vi "Find Path.vi"(8 "error in":errorcluster, 9 "end":string, 10 "start":string, 11 "FlexWorktable in":refnum<class "FlexWorktable.lvclass">) -> (0 "error out":errorcluster, 1 "Point Names":string[](array[string]), 2 "Points":refnum<class "Vec3d.lvclass">[](array[class]), 3 "FlexWorktable out":refnum<class "FlexWorktable.lvclass">)   [LabVIEW 2024]
uses:
  Vec3d Class/Vec3d.lvclass
  FlexWorktable/FlexWorktable.lvclass
  Node.ctl
  fd1d9aa2-fa2c-4f05-b8b8-dc46fe165a2d.vi
  c3290523-0369-4e35-a41e-cda71a30bf11.vi
  852f93a0-a655-4212-b043-5cd013f93269.vi
  5b83d3e8-932b-40b1-bf24-38bcf14b1dea.vi
  <vilib>/Comparison/Equal/Equal Functor/Equal Functor.lvclass
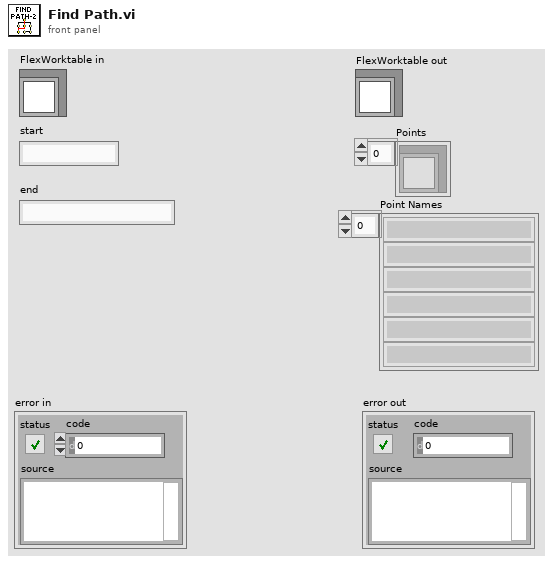
[diagram p1: front panel]
types:
  T1 = typedef "Node.ctl" = cluster{"distance":dbl, "visited":bool, "path to":i32[], "neighbors":i32[], "name":string, "id":i32}
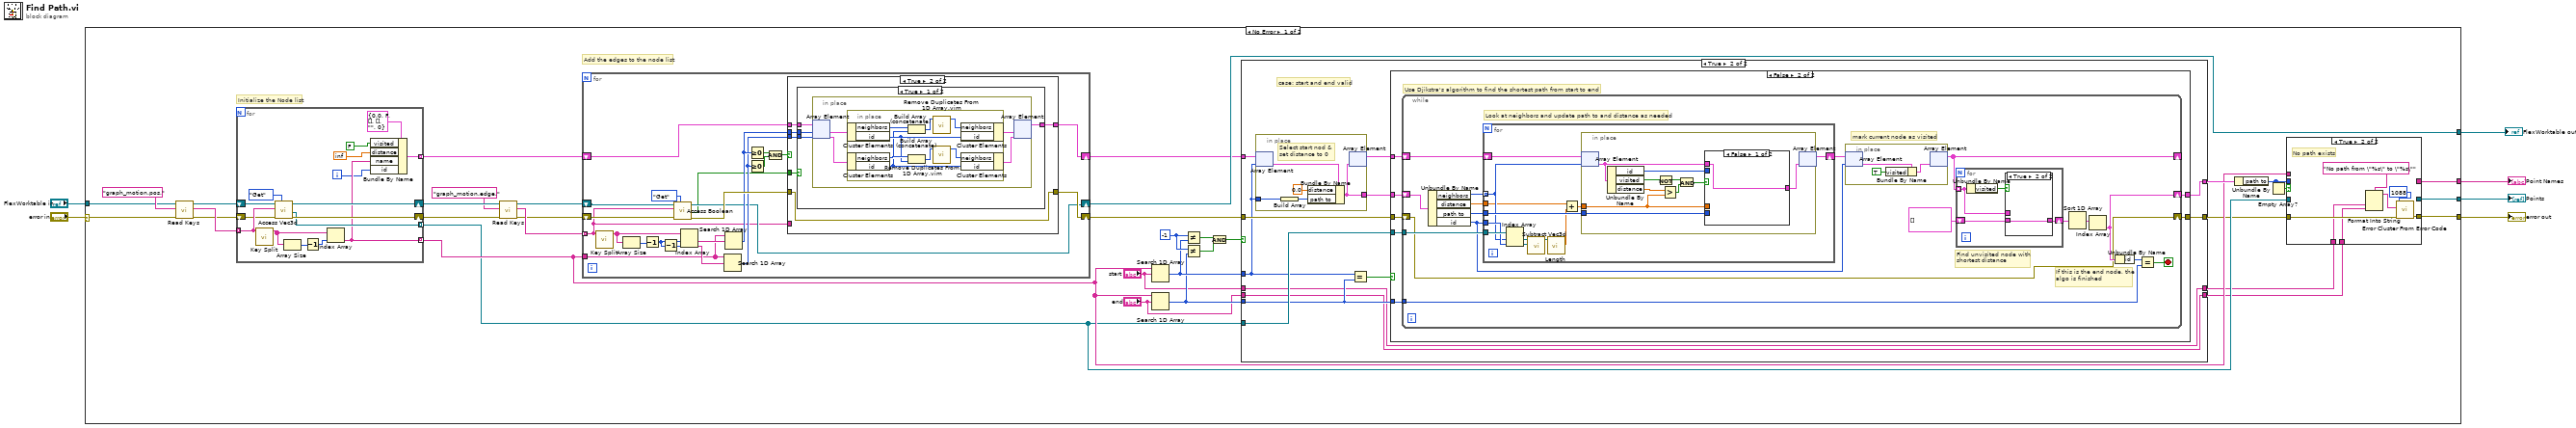
[diagram p0: block diagram]
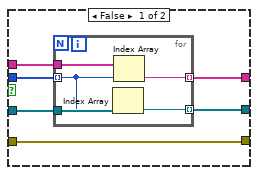
[diagram p2: hidden frame]
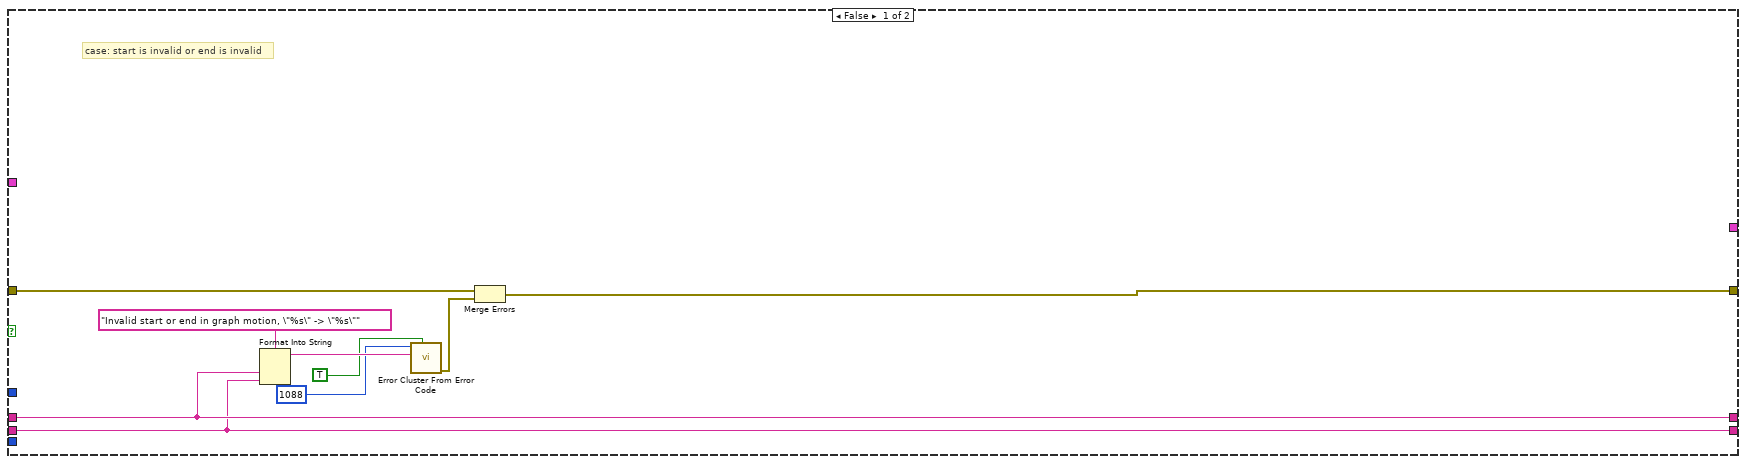
[diagram p3: hidden frame]
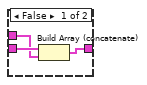
[diagram p5: hidden frame]
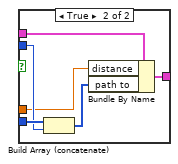
[diagram p6: hidden frame]
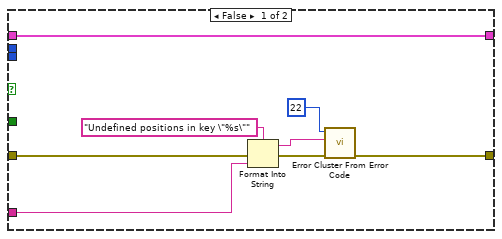
[diagram p7: hidden frame]
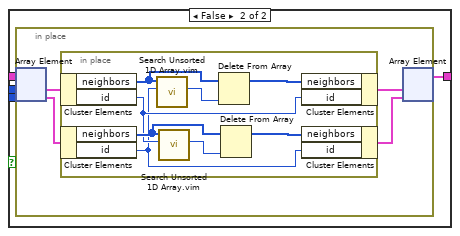
[diagram p8: hidden frame]
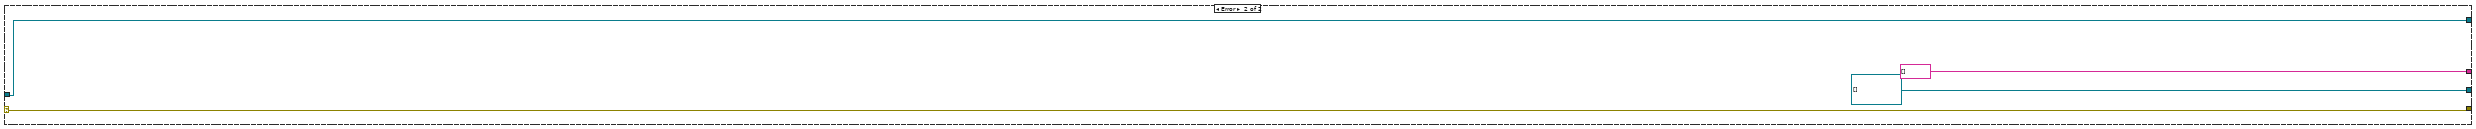
[diagram p9: hidden frame]
diagram:
  n1 = case shown="No Error" "error in" {
    selector: "error in" -> [w15 w238]
    tunnel: [w19 string[] []] -> w6
    tunnel: [w18 refnum<class "Vec3d.lvclass">[] []] -> w5
    tunnel: [w9 w238] -> w4
    tunnel: [w17 w239] -> w3
    tunnel: "FlexWorktable in" -> [w16 w239]
    frame No Error {
      w30 = -1
      # "Add the edges to the node list"
      # "Initialize the Node list"
      n2 = call-dynamic "Read Keys.vi"("error in (no error)"=w15, "Selector"="graph_motion.pos.", "FlexWorktable in"=w16) -> ("error out"=w38:errorcluster, "Keys"=w40:string[], "FlexWorktable out"=w39:refnum<class "FlexWorktable.lvclass">)  [unwired: 6 in]
      n3 = for {
        tunnel: w40 -> [w231] mode=indexing
        tunnel: [w222] -> w21 mode=indexing
        shift-right: [w229] -> w37
        shift-left: w39 -> [w232]
        shift-right: [w227] -> w36
        shift-left: w38 -> [w228]
        tunnel: [w226] -> w20 mode=indexing
        tunnel: [w220] -> w14 mode=indexing
        i -> [w221]
        n4 = call "Key Split.vi"("Key"=w231) -> ("Key Elements"=w234:string[])  [unwired: 10 in]
        n5 = call-dynamic "Access Vec3d.vi"("Get/Set"=enum16{"Get", "Set"}."Get", "error in (no error)"=w228, "Key"=w231, "FlexWorktable in"=w232) -> ("error out"=w227:errorcluster, "Value out"=w226:refnum<class "Vec3d.lvclass">, "FlexWorktable out"=w229:refnum<class "FlexWorktable.lvclass">)  [unwired: 5 in]
        n6 = Array Size(array=w234) -> (size(s)=w235:i32)
        n7 = Decrement(x=w235) -> (x-1=w233:i32)
        n8 = Index Array(array=w234, index=w233) -> (element=w222:string)
        n9 = Bundle By Name(cluster=T1 {"distance"=0.0, "visited"=FALSE, "path to"=[], "neighbors"=[], "name"="", "id"=0}, "visited"=FALSE, "distance"=inf, "name"=w222, "id"=w221) -> (w220:T1)
      }
      n10 = call-dynamic "Read Keys.vi"("error in (no error)"=w36, "Selector"="graph_motion.edge.", "FlexWorktable in"=w37) -> ("error out"=w32:errorcluster, "Keys"=w33:string[], "FlexWorktable out"=w34:refnum<class "FlexWorktable.lvclass">)  [unwired: 6 in]
      n11 = for {
        tunnel: w33 -> [w152] mode=indexing
        tunnel: w21 -> [w167]
        shift-right: [w154] -> w17
        shift-left: w34 -> [w166]
        shift-right: [w160] -> w31
        shift-left: w32 -> [w165]
        shift-right: [w162] -> w13
        shift-left: w14 -> [w163]
        n12 = call "Key Split.vi"("Key"=w152) -> ("Key Elements"=w172:string[])  [unwired: 10 in]
        n13 = Array Size(array=w172) -> (size(s)=w173:i32)
        n14 = Decrement(x=w173) -> (x-1=w171:i32)
        n15 = Decrement(x=w171) -> (x-1=w170:i32)
        n16 = call-dynamic "Access Boolean.vi"("Get/Set"=enum16{"Get", "Set"}."Get", "error in (no error)"=w165, "Key"=w152, "FlexWorktable in"=w166) -> ("error out"=w161:errorcluster, "Value out"=w153:bool, "FlexWorktable out"=w154:refnum<class "FlexWorktable.lvclass">)  [unwired: 5 in]
        n17 = Index Array(array=w172, index #1=w171, index #2=w170) -> (element #1=w169:string, element #2=w168:string)
        n18 = Search 1D Array(1D array=w167, element=w168) -> (index of element=w158:i32)  [unwired: 1 in]
        n19 = Search 1D Array(1D array=w167, element=w169) -> (index of element=w159:i32)  [unwired: 1 in]
        n20 = Greater Or Equal To 0?(x=w159) -> (x >= 0?=w157:bool)
        n21 = Greater Or Equal To 0?(x=w158) -> (x >= 0?=w156:bool)
        n22 = Compound Arithmetic op=AND(w157, w156) -> (w155:bool)
        n23 = case shown="True" w155 {
          tunnel: w163 -> [w181 w187]
          tunnel: [w181 w186] -> w162
          tunnel: w158 -> [_ w185]
          tunnel: w159 -> [_ w184]
          tunnel: w161 -> [w175 w183]
          tunnel: [w180 w183] -> w160
          tunnel: w153 -> [_ w182]
          tunnel: w152 -> [w176 _]
          frame False {
            n24 = Format Into String(format string="Undefined positions in key \"%s\"", error in=w175, w176) -> (resulting string=w178:string, error out=w174:errorcluster)  [unwired: 1 in]
            n25 = call <vilib>:"Error Cluster From Error Code.vi"("error in (no error)"=w174, "error message (\"\")"=w178, "error code (0)"=22) -> ("error out"=w180:errorcluster)  [unwired: 6 in]
          }
          frame True {
            n26 = case shown="True" w182 {
              tunnel: w187 -> [w191 w207]
              tunnel: [w190 w206] -> w186
              tunnel: w185 -> [w189 w205]
              tunnel: w184 -> [w188 w204]
              frame True {
                n27 = in-place {
                  n28 = in-place-array #1(w191, w188, w189) -> (w195:T1, w194:T1)
                  n29 = in-place {
                    n30 = in-place-cluster #2(w195) -> ("neighbors"=w203:i32[], "id"=w201:i32)
                    n31 = in-place-cluster #3(w194) -> ("neighbors"=w202:i32[], "id"=w200:i32)
                    n32 = Build Array (concatenate)(w203, w200) -> (w199:i32[])
                    n33 = Build Array (concatenate)(w202, w201) -> (w197:i32[])
                    n34 = call "Remove Duplicates From 1D Array.vim"("array"=w199) -> ("array with duplicates removed"=w198:i32[])  [unwired: 10 in]
                    n35 = call "Remove Duplicates From 1D Array.vim"("array"=w197) -> ("array with duplicates removed"=w196:i32[])  [unwired: 10 in]
                    n36 = in-place-cluster #2("neighbors"=w198, "id"=w201) -> (w193:T1)
                    n37 = in-place-cluster #3("neighbors"=w196, "id"=w200) -> (w192:T1)
                  }
                  n38 = in-place-array #1(w193, w192) -> (w190:T1[])  [unwired: 2 out]
                }
              }
              frame False {
                n39 = in-place {
                  n40 = in-place-array #4(w207, w204, w205) -> (w211:T1, w210:T1)
                  n41 = in-place {
                    n42 = in-place-cluster #5(w211) -> ("neighbors"=w219:i32[], "id"=w213:i32)
                    n43 = in-place-cluster #6(w210) -> ("neighbors"=w215:i32[], "id"=w212:i32)
                    n44 = call "Search Unsorted 1D Array.vim"("element"=w212, "unsorted 1D array"=w219) -> ("index of element"=w217:i32)  [unwired: 9 in]
                    n45 = call "Search Unsorted 1D Array.vim"("element"=w213, "unsorted 1D array"=w215) -> ("index of element"=w216:i32)  [unwired: 9 in]
                    n46 = Delete From Array(array=w219, index=w217) -> (array with subset deleted=w218:i32[])  [unwired: 1 in, 1 out]
                    n47 = Delete From Array(array=w215, index=w216) -> (array with subset deleted=w214:i32[])  [unwired: 1 in, 1 out]
                    n48 = in-place-cluster #5("neighbors"=w218, "id"=w213) -> (w209:T1)
                    n49 = in-place-cluster #6("neighbors"=w214, "id"=w212) -> (w208:T1)
                  }
                  n50 = in-place-array #4(w209, w208) -> (w206:T1[])  [unwired: 2 out]
                }
              }
            }
          }
        }
      }
      n51 = Search 1D Array(1D array=w21, element="start") -> (index of element=w29:i32)  [unwired: 1 in]
      n52 = Search 1D Array(1D array=w21, element="end") -> (index of element=w28:i32)  [unwired: 1 in]
      n53 = Not Equal?(x=w30, y=w29) -> (x != y?=w25:bool)
      n54 = Not Equal?(x=w30, y=w28) -> (x != y?=w23:bool)
      n55 = And(x=w25, y=w23) -> (x .and. y?=w24:bool)
      n56 = case shown="True" w24 {
        tunnel: w29 -> [_ w71]
        tunnel: w31 -> [w64 w80]
        tunnel: w20 -> [_ w79]
        tunnel: w28 -> [_ w75]
        tunnel: "start" -> [w61 w70]
        tunnel: "end" -> [w60 w69]
        tunnel: [w62 w78] -> w10
        tunnel: [_ w76] -> w22
        tunnel: w13 -> [_ w73]
        tunnel: [w61 w70] -> w8
        tunnel: [w60 w69] -> w7
        frame False {
          # "case: start is invalid or end is invalid"
          n57 = Format Into String(format string="Invalid start or end in graph motion, \"%s\" -> \"%s\"", w61, w60) -> (resulting string=w67:string)  [unwired: 2 in, 1 out]
          n58 = call <vilib>:"Error Cluster From Error Code.vi"("show call chain? (False)"=TRUE, "error message (\"\")"=w67, "error code (0)"=1088) -> ("error out"=w63:errorcluster)  [unwired: 6 in]
          n59 = Merge Errors(w64, w63) -> (w62:errorcluster)
        }
        frame True {
          # "case: start and end valid"
          n60 = in-place {
            in-place-border: [w81] -> w77
            in-place-border: w71 -> [w83]
            # "Select start nod & \nset distance to 0"
            n61 = in-place-array #7(w73, w71) -> (w82:T1)
            n62 = Build Array(w83) -> (w84:i32[])
            n63 = Bundle By Name(cluster=w82, "distance"=0.0, "path to"=w84) -> (w81:T1)
            n64 = in-place-array #7(w81) -> (w72:T1[])  [unwired: 1 out]
          }
          n65 = Equal?(x=w71, y=w75) -> (x = y?=w74:bool)
          n66 = case shown="False" w74 {
            tunnel: w80 -> [w86 w94]
            tunnel: w79 -> [_ w93]
            tunnel: w75 -> [_ w92]
            tunnel: [w86 w91] -> w78
            tunnel: w72 -> [_ w90]
            tunnel: w77 -> [w87 w89]
            tunnel: [w87 w88] -> w76
            frame True {
              # "Start and end are the same point"
            }
            frame False {
              # "Use Djikstra's algorithm to find the shortest path from start to end"
              n67 = while {
                shift-right: [w95] -> w91
                shift-left: w94 -> [w95]
                tunnel: w93 -> [w106]
                tunnel: w92 -> [w98]
                shift-right: [w97] -> w88
                shift-left: w89 -> [w111]
                shift-right: [w103] -> _
                shift-left: w90 -> [w109]
                stop <- w96 stop-if-true
                # "If this is the end node, the algo is finished"
                # "Find unvisited node with\nshortest distance"
                # "mark current node as visited"
                # "Look at neighbors and update path to and distance as needed"
                n68 = Unbundle By Name(w111) -> ("neighbors"=w110:i32[], "distance"=w108:dbl, "path to"=w107:i32[], "id"=w104:i32)
                n69 = for {
                  tunnel: w110 -> [w127] mode=indexing
                  tunnel: w108 -> [w125]
                  tunnel: w107 -> [w129]
                  tunnel: w104 -> [w133]
                  tunnel: w106 -> [w134]
                  shift-right: [w123] -> w105
                  shift-left: w109 -> [w128]
                  n70 = Index Array(array=w134, index #1=w127, index #2=w133) -> (element #1=w131:refnum<class "Vec3d.lvclass">, element #2=w130:refnum<class "Vec3d.lvclass">)
                  n71 = call "Subtract Vec3d.vi"("Vec3d in 2"=w130, "Vec3d in 1"=w131) -> ("Vec3d Class out"=w132:refnum<class "Vec3d.lvclass">)  [unwired: 8 in, 1 out]
                  n72 = call-dynamic "Length.vi"("Vec3d in"=w132) -> ("Length"=w126:dbl)  [unwired: 8 in, 2 out]
                  n73 = Add(x=w125, y=w126) -> (x+y=w124:dbl)
                  n74 = in-place {
                    in-place-border: w129 -> [w139]
                    in-place-border: w124 -> [w135]
                    n75 = in-place-array #8(w128, w127) -> (w137:T1)
                    n76 = Unbundle By Name(w137) -> ("id"=w138:i32, "visited"=w144:bool, "distance"=w143:dbl)
                    n77 = Not(x=w144) -> (.not. x?=w140:bool)
                    n78 = Greater?(x=w143, y=w135) -> (0:w141:bool)
                    n79 = And(x=w140, y=w141) -> (x .and. y?=w142:bool)
                    n80 = case shown="False" w142 {
                      tunnel: w137 -> [w145 w151]
                      tunnel: w135 -> [_ w147]
                      tunnel: w139 -> [_ w150]
                      tunnel: w138 -> [_ w149]
                      tunnel: [w145 w146] -> w136
                      frame False {
                      }
                      frame True {
                        n81 = Build Array (concatenate)(w150, w149) -> (w148:i32[])
                        n82 = Bundle By Name(cluster=w151, "distance"=w147, "path to"=w148) -> (w146:T1)
                      }
                    }
                    n83 = in-place-array #8(w136) -> (w123:T1[])  [unwired: 1 out]
                  }
                }
                n84 = in-place {
                  n85 = in-place-array #9(w105, w104) -> (w122:T1)
                  n86 = Bundle By Name(cluster=w122, "visited"=TRUE) -> (w120:T1)
                  n87 = in-place-array #9(w120) -> (w103:T1[])  [unwired: 1 out]
                }
                n88 = for {
                  tunnel: w103 -> [w112] mode=indexing
                  shift-right: [w113] -> w101
                  shift-left: T1[] [] -> [w114]
                  n89 = Unbundle By Name(w112) -> ("visited"=w115:bool)
                  n90 = case shown="True" w115 {
                    tunnel: w114 -> [w118 w119]
                    tunnel: [w116 w119] -> w113
                    tunnel: w112 -> [w117 _]
                    frame False {
                      n91 = Build Array (concatenate)(w118, w117) -> (w116:T1[])
                    }
                    frame True {
                    }
                  }
                }
                n92 = Sort 1D Array(array=w101) -> (sorted array=w100:T1[])
                n93 = Index Array(array=w100) -> (element=w97:T1)  [unwired: 1 in]
                n94 = Unbundle By Name(w97) -> ("id"=w99:i32)
                n95 = Equal?(x=w99, y=w98) -> (x = y?=w96:bool)
              }
            }
          }
        }
      }
      n96 = Unbundle By Name(w22) -> ("path to"=w12:i32[])
      n97 = Empty Array?(array=w12) -> (empty?=w11:bool)
      n98 = case shown="True" w11 {
        tunnel: w12 -> [w47 _]
        tunnel: w21 -> [w46 _]
        tunnel: w20 -> [w45 _]
        tunnel: [w44 _] -> w19
        tunnel: [w43 _] -> w18
        tunnel: w10 -> [w42 w56]
        tunnel: [w42 w55] -> w9
        tunnel: w8 -> [_ w54]
        tunnel: w7 -> [_ w53]
        frame False {
          n99 = for {
            tunnel: w47 -> [w50] mode=indexing
            tunnel: w46 -> [w52]
            tunnel: w45 -> [w51]
            tunnel: [w49] -> w44 mode=indexing
            tunnel: [w48] -> w43 mode=indexing
            n100 = Index Array(array=w51, index=w50) -> (element=w48:refnum<class "Vec3d.lvclass">)
            n101 = Index Array(array=w52, index=w50) -> (element=w49:string)
          }
        }
        frame True {
          # "No path exists"
          n102 = Format Into String(format string="No path from \"%s\" to \"%s\"", w54, w53) -> (resulting string=w59:string)  [unwired: 2 in, 1 out]
          n103 = call <vilib>:"Error Cluster From Error Code.vi"("error in (no error)"=w56, "error message (\"\")"=w59, "error code (0)"=1088) -> ("error out"=w55:errorcluster)  [unwired: 6 in]
        }
      }
    }
    frame Error {
    }
  }
  "error out" <- w4
  "Point Names" <- w6
  "Points" <- w5
  "FlexWorktable out" <- w3
